vi "Battery Voltage.vi"() -> (0 "New Motor Signal":dbl)   [LabVIEW 2012]
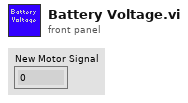
[diagram p1: front panel]
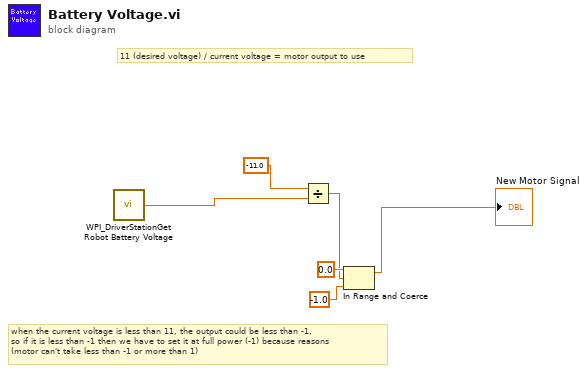
[diagram p0: block diagram]
diagram:
  # "when the current voltage is less than 11, the output could be less than -1,\nso if it is less than -1 then we have to set it at full power (-1) because reasons\n(motor can't take less than -1 or more than 1)"
  # "11 (desired voltage) / current voltage = motor output to use"
  n1 = call <vilib>:"WPI_DriverStationGet Robot Battery Voltage.vi"() -> ("robot battery voltage"=w1:dbl)  [unwired: 14 in, 1 out]
  n2 = Divide(x=-11.0, y=w1) -> (x/y=w3:dbl)
  n3 = In Range and Coerce(upper limit=0.0, x=w3, lower limit=-1.0) -> (coerced(x)=→"New Motor Signal":dbl)  [unwired: 1 out]
